vi "Control Globals.vi"() -> ()   [LabVIEW 2025]
panel:
  in  "Terminate All Button":refnum<k7>
  in  "Sequence Files ComboBox":refnum<k7>
  in  "Sequences ComboBox":refnum<k7>
  in  "Open Sequence File Button":refnum<k7>
  in  "Close Sequence File Button":refnum<k7>
  in  "Entry Point 1 Button":refnum<k7>
  in  "Entry Point 2 Button":refnum<k7>
  in  "Run Selected Sequence Button":refnum<k7>
  in  "Executions ComboBox":refnum<k7>
  in  "Execution View":refnum<k7>
  in  "Report Viewer":refnum<k7>
  in  "Close Executions Button":refnum<k7>
  in  "Break/Resume Button":refnum<k7>
  in  "Terminate/Restart Button":refnum<k7>
  in  "Application Manager":refnum<k7>
  in  "SequenceFileView Manager":refnum<k7>
  in  "ExecutionView Manager":refnum<k7>
  in  "Quit Application Event":refnum<user-event>
  in  "Top level VI":refnum<vi>
  in  "TestStand Engine":refnum<k7>
  in  "Event Callback":refnum<k27>
  # "Other References"
  # "Manager Controls"
  # "Visible Controls"
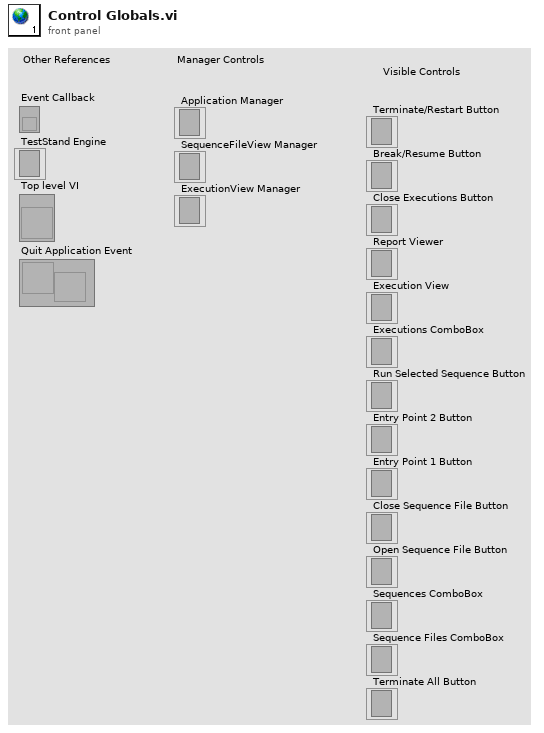
[diagram p1: front panel]
diagram:
